vi "String - Convert IP Address Byte Array to String.vi"(11 "Array of Bytes":u8[](array[numeric])) -> (3 "IP Address String":string)   [LabVIEW 2020]
doc: "Converts an array of 4 bytes, representing an IP address, into a string."
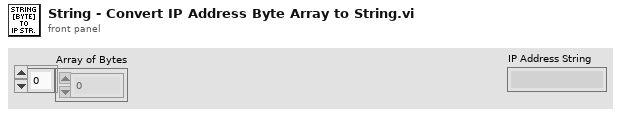
[diagram p1: front panel]
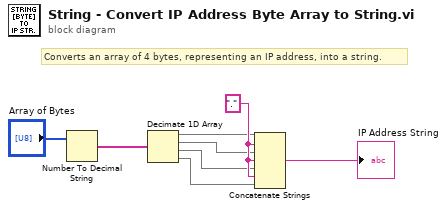
[diagram p0: block diagram]
diagram:
  w7 = "."
  # "Converts an array of 4 bytes, representing an IP address, into a string."
  n1 = Number To Decimal String(number="Array of Bytes") -> (decimal integer string=w2:string[])  [unwired: 1 in]
  n2 = Decimate 1D Array(w2) -> (w3:string[], w4:string[], w5:string[], w6:string[])
  n3 = Concatenate Strings(w3, w7, w4, w7, w5, w7, w6) -> (→"IP Address String":string)
